vi "MJG_UDPtester_v1.vi"() -> ()   [LabVIEW 2016]
panel:
  out "cmdArray":sgl[](array[numeric])
  in  "stop":bool
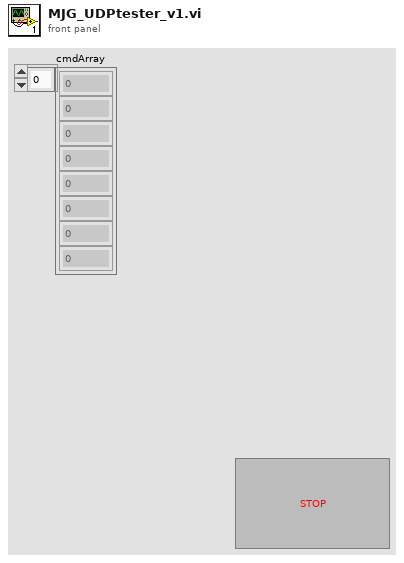
[diagram p1: front panel]
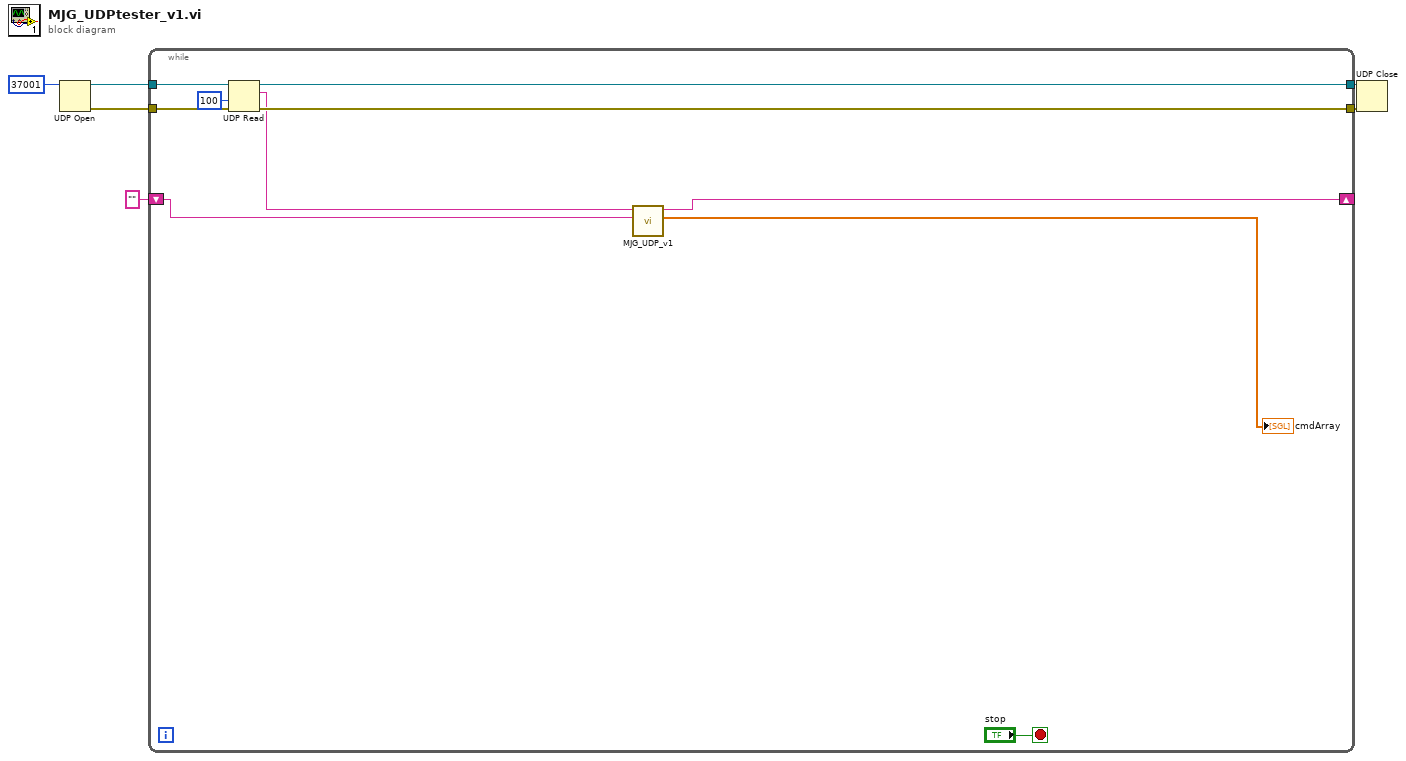
[diagram p0: block diagram]
diagram:
  n1 = UDP Open(11:u16 37001 ("port")) -> (port=w5:refnum<k16>, 0:w4:errorcluster)  [unwired: 4 in, 1 out]
  n2 = while {
    tunnel: w5 -> [w14]
    tunnel: w4 -> [w13]
    tunnel: [w12] -> w3
    tunnel: [w11] -> w2
    shift-right: [w7] -> _
    shift-left: "" ("data out") -> [w8]
    stop <- "stop" stop-if-true
    n3 = UDP Read(connection ID=w14, timeout ms (25000)=100, 8:w13) -> (data out=w9:string, error out=w11:errorcluster, 3:w12:refnum<k16>)  [unwired: 1 in, 2 out]
    n4 = call "MJG_UDP_v1.vi"("prev string"=w8, "string received"=w9) -> ("cmdArray"=→"cmdArray":sgl[], "string out"=w7:string)  [unwired: 8 in]
  }
  n5 = UDP Close(connection ID=w3, 8:w2) -> ()  [unwired: 2 out]
